vi "createPubDataEvents.vi"(8 "error in (no error)":errorcluster, 11 "UserEvents in":refnum<class "UserEvents.lvclass">) -> (0 "error out":errorcluster, 3 "UserEvents out":refnum<class "UserEvents.lvclass">)   [LabVIEW 2015, in "UserEvents.lvclass"]
uses:
  UserEvents.lvclass
  Typedefs/StateSelector.ctl
  Typedefs/InputData.ctl
  Typedefs/ForceDemand.ctl
  <userlib>/Common/Devices/DistanceGauge/Typedefs/Distance Data.ctl
  Typedefs/OutputData.ctl
  Typedefs/ControllerData.ctl
  Typedefs/TestStatus.ctl
  Typedefs/StiffnessData.ctl
  UserEvents.lvclass/UserEvents.ctl
  Typedefs/M1M3SSSTypedefs.lvlib
  <userlib>/Common/Devices/DistanceGauge/DistanceGauge.lvlib
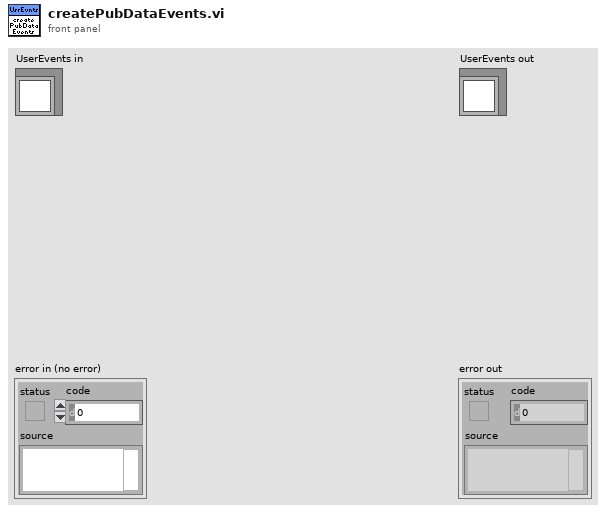
[diagram p1: front panel]
types:
  T1 = typedef "M1M3SSSTypedefs.lvlib/StiffnessData.ctl" = cluster{"Distance Measured":dbl[unit][], "Force Measured":dbl[unit][]}
  T2 = typedef "M1M3SSSTypedefs.lvlib/TestStatus.ctl" = cluster{"activeCycle":u32, "activeProfileStep":u32, "demandedCycles":u32, "demandedProfileSteps":u32}
  T3 = typedef "M1M3SSSTypedefs.lvlib/ControllerData.ctl" = cluster{"Force Demand":T4, "Force Error":T4}
  T4 = typedef "M1M3SSSTypedefs.lvlib/ForceDemand.ctl" = dbl[unit]
  T5 = typedef "M1M3SSSTypedefs.lvlib/OutputData.ctl" = cluster{"Ramp Output":u16}
  T6 = typedef "M1M3SSSTypedefs.lvlib/InputData.ctl" = cluster{"Force Measured":T4, "Distance Data":T7}
  T7 = typedef "DistanceGauge.lvlib/Distance Data.ctl" = cluster{"Distance Measured 1":dbl[unit], "Distance Measured 2":dbl[unit]}
  T8 = typedef "M1M3SSSTypedefs.lvlib/StateSelector.ctl" = enum16{"FaultState", "OffState", "RampingUpPressurePState", "RampingUpPressureSTState", "StandbyState", "StoppedState", "WaitingForSettledPState", "WaitingForSettledSTState"}
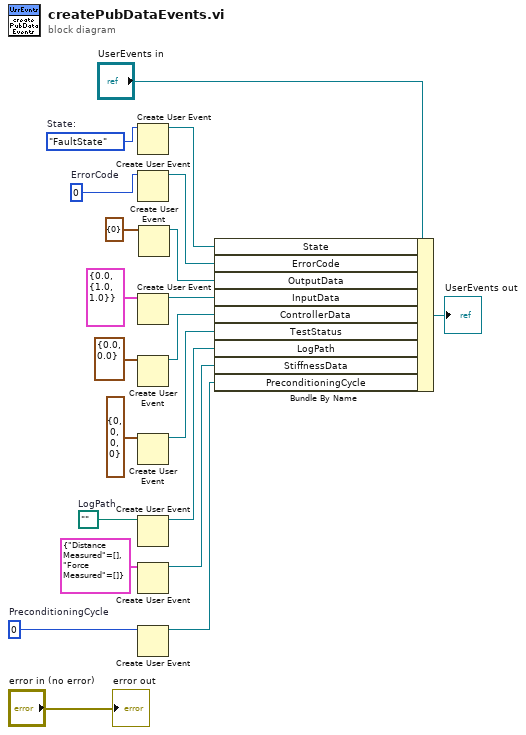
[diagram p0: block diagram]
diagram:
  w2 = u32 0  # PreconditioningCycle
  w6 = path ""  # LogPath
  w17 = 0  # ErrorCode
  w18 = StateSelector."FaultState"  # State:
  n1 = Create User Event(user event datatype=w18) -> (user event=w16:refnum<user-event>)  [unwired: 1 in, 1 out]
  n2 = Create User Event(user event datatype=w17) -> (user event=w15:refnum<user-event>)  [unwired: 1 in, 1 out]
  n3 = Create User Event(user event datatype=T6 {"Force Measured"=0.0, "Distance Data"={"Distance Measured 1"=1.0, "Distance Measured 2"=1.0}} ("Input Data")) -> (user event=w13:refnum<user-event>)  [unwired: 1 in, 1 out]
  n4 = Create User Event(user event datatype=T3 {"Force Demand"=0.0, "Force Error"=0.0} ("Controller Data")) -> (user event=w9:refnum<user-event>)  [unwired: 1 in, 1 out]
  n5 = Create User Event(user event datatype=T2 {"activeCycle"=0, "activeProfileStep"=0, "demandedCycles"=0, "demandedProfileSteps"=0} ("TestStatus")) -> (user event=w7:refnum<user-event>)  [unwired: 1 in, 1 out]
  n6 = Create User Event(user event datatype=w6) -> (user event=w5:refnum<user-event>)  [unwired: 1 in, 1 out]
  n7 = Create User Event(user event datatype=T1 {"Distance Measured"=[], "Force Measured"=[]} ("output cluster")) -> (user event=w3:refnum<user-event>)  [unwired: 1 in, 1 out]
  n8 = Create User Event(user event datatype=w2) -> (user event=w1:refnum<user-event>)  [unwired: 1 in, 1 out]
  n9 = Create User Event(user event datatype=T5 {"Ramp Output"=0} ("Output Data")) -> (user event=w11:refnum<user-event>)  [unwired: 1 in, 1 out]
  n10 = Bundle By Name(cluster="UserEvents in", "State"=w16, "ErrorCode"=w15, "OutputData"=w11, "InputData"=w13, "ControllerData"=w9, "TestStatus"=w7, "LogPath"=w5, "StiffnessData"=w3, "PreconditioningCycle"=w1) -> (→"UserEvents out":refnum<class "UserEvents.lvclass">)
  "error out" <- "error in (no error)"
